vi "OnOff Test Demo.vi"() -> ()   [LabVIEW 2012]
uses:
  LabVIEW/user.lib/SpectralRadar.llb/set Spectrum Output.vi
  LabVIEW/user.lib/SpectralRadar.llb/display Data 2D.vi
  LabVIEW/user.lib/SpectralRadar.llb/set Scan Output.vi
  LabVIEW/user.lib/SpectralRadar.llb/set Apodized Spectrum Output.vi
  LabVIEW/user.lib/SpectralRadar.llb/OCT Device.lvclass
  LabVIEW/user.lib/SpectralRadar.llb/Probe.lvclass
  LabVIEW/user.lib/SpectralRadar.llb/Processing.lvclass
  LabVIEW/user.lib/SpectralRadar.llb/Raw Data.lvclass
  LabVIEW/user.lib/SpectralRadar.llb/Data.lvclass
  LabVIEW/user.lib/SpectralRadar.llb/Scan Pattern.lvclass
panel:
  in  "AScans 2":i32=512
  in  "stop":bool
  out "B-Scan Data":dbl[][](graph)
  out "Spectral Data":dbl[][](graph)
  in  "AScans":i32=512
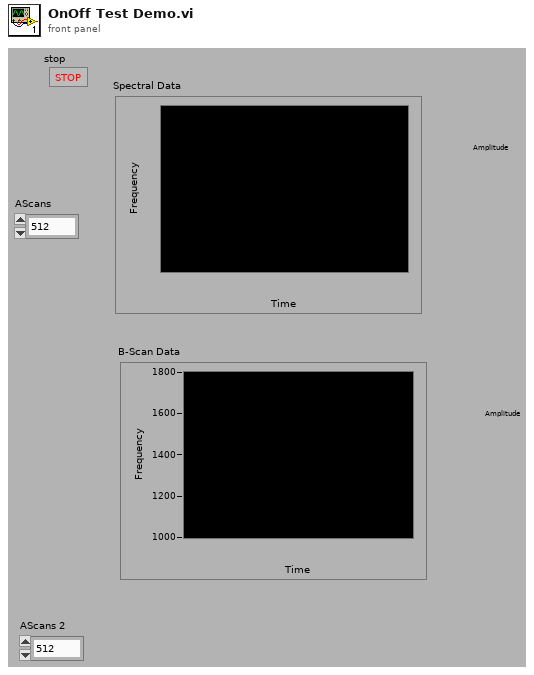
[diagram p1: front panel]
types:
  T1 = enum16{"Asynchronous Continuous", "Asynchronous Finite", "Synchronous"}
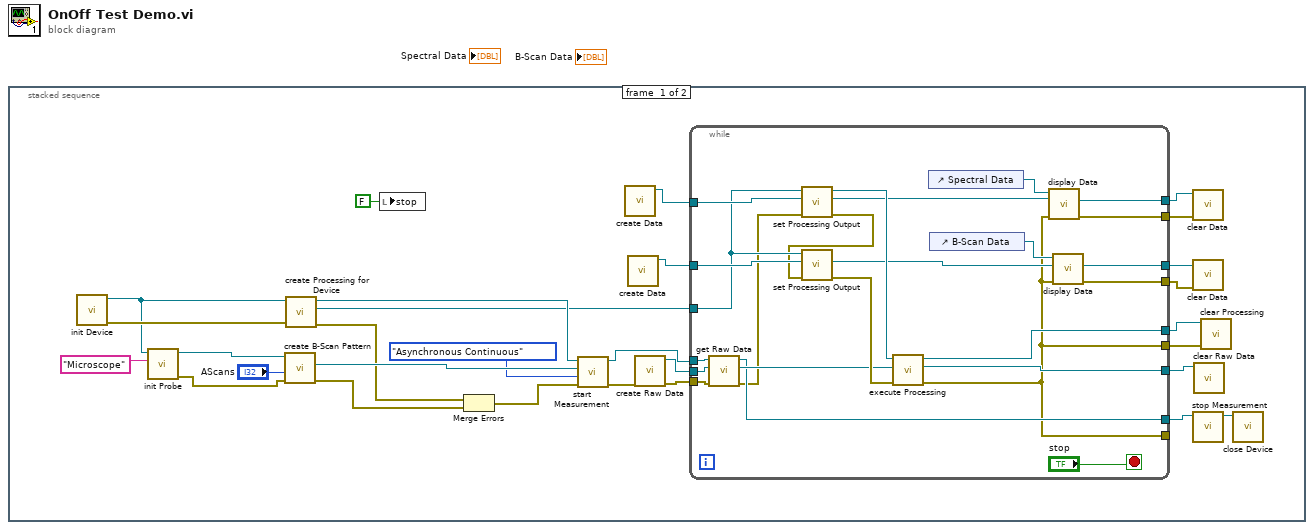
[diagram p0: block diagram]
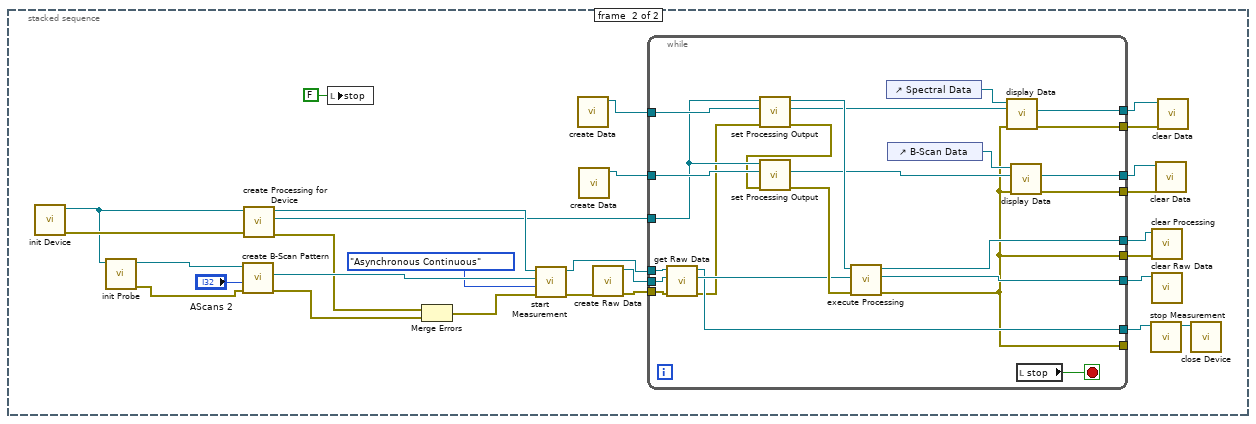
[diagram p2: hidden frame]
diagram:
  n1 = stacked-sequence {
    frame #0 {
      n2 = call "init Device.vi"() -> ("error out"=w28:errorcluster, "OCTDevice"=w14:refnum<class "OCT Device.lvclass">)  [unwired: 6 in]
      n3 = call "init Probe.vi"("Probe"="Microscope", "OCT Device"=w14) -> ("error out"=w13:errorcluster, "GalvoControl"=w27:refnum<class "Probe.lvclass">)  [unwired: 4 in]
      n4 = call "create B-Scan Pattern.vi"("error in (no error)"=w13, "AScans"="AScans", "Probe"=w27) -> ("error out"=w23:errorcluster, "Scan Pattern"=w25:refnum<class "Scan Pattern.lvclass">)  [unwired: 3 in, 1 out]
      n5 = call "create Processing for Device.vi"("error in (no error)"=w28, "OCTDevice"=w14) -> ("error out"=w21:errorcluster, "Processing"=w16:refnum<class "Processing.lvclass">, "OCTDevice"=w17:refnum<class "OCT Device.lvclass">)  [unwired: 3 in]
      n6 = local write "stop"(FALSE ("stop")) -> ()
      n7 = Merge Errors(w21, w23) -> (w22:errorcluster)
      n8 = call "start Measurement.vi"("error in (no error)"=w22, "Acquisition Type"=T1."Asynchronous Continuous", "Scan Pattern"=w25, "OCTDevice"=w17) -> ("error out"=w19:errorcluster, "OCTDevice"=w10:refnum<class "OCT Device.lvclass">)  [unwired: 1 in, 1 out]
      n9 = call "create Data.vi"() -> ("Data"=w2:refnum<class "Data.lvclass">)  [unwired: 6 in, 1 out]
      n10 = call "create Data.vi"() -> ("Data"=w1:refnum<class "Data.lvclass">)  [unwired: 6 in, 1 out]
      n11 = call "create Raw Data.vi"("error in (no error)"=w19) -> ("error out"=w18:errorcluster, "Raw Data"=w20:refnum<class "Raw Data.lvclass">)  [unwired: 5 in]
      n12 = while {
        tunnel: w20 -> [w52]
        tunnel: w10 -> [w53]
        tunnel: w18 -> [w51]
        tunnel: w16 -> [w48]
        tunnel: w1 -> [w50]
        tunnel: w2 -> [w49]
        tunnel: [w39] -> w15
        tunnel: [w38] -> w8
        tunnel: [w37] -> w4
        tunnel: [w36] -> w6
        tunnel: [w35] -> w3
        tunnel: [w34] -> w5
        tunnel: [w33] -> w12
        tunnel: [w31] -> w7
        tunnel: [w31] -> _
        stop <- "stop" stop-if-true
        n13 = call "get Raw Data.vi"("error in (no error)"=w51, "RawData in"=w52, "OCTDevice in"=w53) -> ("error out"=w32:errorcluster, "RawData out"=w44:refnum<class "Raw Data.lvclass">, "OCTDevice out"=w33:refnum<class "OCT Device.lvclass">)  [unwired: 2 in]
        n14 = call-poly "set Processing Output.vi"("error in (no error)"=w32, "Data"=w49, "Processing"=w48) -> ("error out"=w46:errorcluster, "Data"=w42:refnum<class "Data.lvclass">, "Processing"=w47:refnum<class "Processing.lvclass">)  [unwired: 2 in]
        n15 = call-poly "set Processing Output.vi"("error in (no error)"=w46, "Data"=w50, "Processing"=w48) -> ("error out"=w45:errorcluster, "Data"=w40:refnum<class "Data.lvclass">)  [unwired: 2 in, 1 out]
        n16 = call "execute Processing.vi"("error in (no error)"=w45, "Raw Data"=w44, "Processing"=w47) -> ("error out"=w31:errorcluster, "Raw Data"=w39:refnum<class "Raw Data.lvclass">, "Processing"=w38:refnum<class "Processing.lvclass">)  [unwired: 2 in]
        n17 = control-ref of="Spectral Data"() -> (w43:refnum<vi>)
        n18 = control-ref of="B-Scan Data"() -> (w41:refnum<vi>)
        n19 = call-poly "display Data.vi"("error in (no error)"=w31, "Data in"=w42, "IntGraph Refnum"=w43) -> ("error out"=w34:errorcluster, "Data out"=w36:refnum<class "Data.lvclass">)  [unwired: 2 in, 1 out]
        n20 = call-poly "display Data.vi"("error in (no error)"=w31, "Data in"=w40, "IntGraph Refnum"=w41) -> ("error out"=w35:errorcluster, "Data out"=w37:refnum<class "Data.lvclass">)  [unwired: 2 in, 1 out]
      }
      n21 = call "clear Data.vi"("error in (no error)"=w5, "Data"=w6) -> ()  [unwired: 5 in, 1 out]
      n22 = call "clear Data.vi"("error in (no error)"=w3, "Data"=w4) -> ()  [unwired: 5 in, 1 out]
      n23 = call "stop Measurement.vi"("OCTDevice"=w12) -> ("OCTDevice"=w11:refnum<class "OCT Device.lvclass">)  [unwired: 5 in, 1 out]
      n24 = call "clear Raw Data.vi"("Raw Data"=w15) -> ()  [unwired: 6 in, 1 out]
      n25 = call "clear Processing.vi"("error in (no error)"=w7, "Processing"=w8) -> ()  [unwired: 5 in, 1 out]
      n26 = call "close Device.vi"("OCTDevice"=w11) -> ()  [unwired: 6 in, 1 out]
    }
    frame #1 {
      n27 = call "init Device.vi"() -> ("error out"=w81:errorcluster, "OCTDevice"=w67:refnum<class "OCT Device.lvclass">)  [unwired: 6 in]
      n28 = call "init Probe.vi"("OCT Device"=w67) -> ("error out"=w66:errorcluster, "GalvoControl"=w80:refnum<class "Probe.lvclass">)  [unwired: 5 in]
      n29 = call "create B-Scan Pattern.vi"("error in (no error)"=w66, "AScans"="AScans 2", "Probe"=w80) -> ("error out"=w76:errorcluster, "Scan Pattern"=w78:refnum<class "Scan Pattern.lvclass">)  [unwired: 3 in, 1 out]
      n30 = call "create Processing for Device.vi"("error in (no error)"=w81, "OCTDevice"=w67) -> ("error out"=w74:errorcluster, "Processing"=w69:refnum<class "Processing.lvclass">, "OCTDevice"=w70:refnum<class "OCT Device.lvclass">)  [unwired: 3 in]
      n31 = local write "stop"(FALSE ("stop")) -> ()
      n32 = Merge Errors(w74, w76) -> (w75:errorcluster)
      n33 = call "start Measurement.vi"("error in (no error)"=w75, "Acquisition Type"=T1."Asynchronous Continuous", "Scan Pattern"=w78, "OCTDevice"=w70) -> ("error out"=w72:errorcluster, "OCTDevice"=w63:refnum<class "OCT Device.lvclass">)  [unwired: 1 in, 1 out]
      n34 = call "create Data.vi"() -> ("Data"=w59:refnum<class "Data.lvclass">)  [unwired: 6 in, 1 out]
      n35 = call "create Data.vi"() -> ("Data"=w58:refnum<class "Data.lvclass">)  [unwired: 6 in, 1 out]
      n36 = call "create Raw Data.vi"("error in (no error)"=w72) -> ("error out"=w71:errorcluster, "Raw Data"=w73:refnum<class "Raw Data.lvclass">)  [unwired: 5 in]
      n37 = while {
        tunnel: w73 -> [w104]
        tunnel: w63 -> [w105]
        tunnel: w71 -> [w103]
        tunnel: w69 -> [w100]
        tunnel: w58 -> [w102]
        tunnel: w59 -> [w101]
        tunnel: [w91] -> w68
        tunnel: [w90] -> w61
        tunnel: [w89] -> w55
        tunnel: [w88] -> w57
        tunnel: [w87] -> w54
        tunnel: [w86] -> w56
        tunnel: [w85] -> w65
        tunnel: [w83] -> w60
        tunnel: [w83] -> _
        stop <- w82 stop-if-true
        n38 = call "get Raw Data.vi"("error in (no error)"=w103, "RawData in"=w104, "OCTDevice in"=w105) -> ("error out"=w84:errorcluster, "RawData out"=w96:refnum<class "Raw Data.lvclass">, "OCTDevice out"=w85:refnum<class "OCT Device.lvclass">)  [unwired: 2 in]
        n39 = call-poly "set Processing Output.vi"("error in (no error)"=w84, "Data"=w101, "Processing"=w100) -> ("error out"=w98:errorcluster, "Data"=w94:refnum<class "Data.lvclass">, "Processing"=w99:refnum<class "Processing.lvclass">)  [unwired: 2 in]
        n40 = call-poly "set Processing Output.vi"("error in (no error)"=w98, "Data"=w102, "Processing"=w100) -> ("error out"=w97:errorcluster, "Data"=w92:refnum<class "Data.lvclass">)  [unwired: 2 in, 1 out]
        n41 = call "execute Processing.vi"("error in (no error)"=w97, "Raw Data"=w96, "Processing"=w99) -> ("error out"=w83:errorcluster, "Raw Data"=w91:refnum<class "Raw Data.lvclass">, "Processing"=w90:refnum<class "Processing.lvclass">)  [unwired: 2 in]
        n42 = control-ref of="Spectral Data"() -> (w95:refnum<vi>)
        n43 = control-ref of="B-Scan Data"() -> (w93:refnum<vi>)
        n44 = call-poly "display Data.vi"("error in (no error)"=w83, "Data in"=w94, "IntGraph Refnum"=w95) -> ("error out"=w86:errorcluster, "Data out"=w88:refnum<class "Data.lvclass">)  [unwired: 2 in, 1 out]
        n45 = call-poly "display Data.vi"("error in (no error)"=w83, "Data in"=w92, "IntGraph Refnum"=w93) -> ("error out"=w87:errorcluster, "Data out"=w89:refnum<class "Data.lvclass">)  [unwired: 2 in, 1 out]
        n46 = local read "stop"() -> (w82:bool)
      }
      n47 = call "stop Measurement.vi"("OCTDevice"=w65) -> ("OCTDevice"=w64:refnum<class "OCT Device.lvclass">)  [unwired: 5 in, 1 out]
      n48 = call "clear Processing.vi"("error in (no error)"=w60, "Processing"=w61) -> ()  [unwired: 5 in, 1 out]
      n49 = call "clear Raw Data.vi"("Raw Data"=w68) -> ()  [unwired: 6 in, 1 out]
      n50 = call "clear Data.vi"("error in (no error)"=w54, "Data"=w55) -> ()  [unwired: 5 in, 1 out]
      n51 = call "clear Data.vi"("error in (no error)"=w56, "Data"=w57) -> ()  [unwired: 5 in, 1 out]
      n52 = call "close Device.vi"("OCTDevice"=w64) -> ()  [unwired: 6 in, 1 out]
    }
  }
